vi "Write serialNumber.vi"(8 "error in (no error)":errorcluster, 10 "serialNumber":string, 11 "CCD in":refnum<class "CCD.lvclass">) -> (0 "error out":errorcluster, 3 "CCD out":refnum<class "CCD.lvclass">)   [LabVIEW 2020, in "horiba.lvlib" / "CCD.lvclass"]
doc: "Sets the device serial after init"
uses:
  CCD.lvclass
  GenericDevice/GenericDevice.lvclass
panel:
  # "Connector Pane"
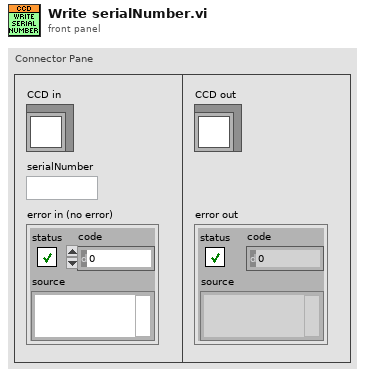
[diagram p1: front panel]
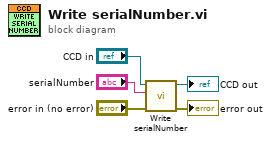
[diagram p0: block diagram]
diagram:
  n1 = call-parent "Write serialNumber.vi"("error in (no error)"="error in (no error)", "serialNumber"="serialNumber", "GenericDevice in"="CCD in") -> ("error out"=→"error out":errorcluster, "GenericDevice out"=→"CCD out":refnum<class "CCD.lvclass">)  [unwired: 7 in]
